vi "create and initialize.vi"(8 "error in":errorcluster, 10 "parameters":variant, 11 "function":T1) -> (0 "error out":errorcluster, 3 "call by reference action":refnum<class "call function by reference.lvclass">)   [LabVIEW 2014, in "call function by reference.lvclass"]
uses:
  call function by reference.lvclass
  function definition.ctl
  call function by reference.lvclass/call function by reference.ctl
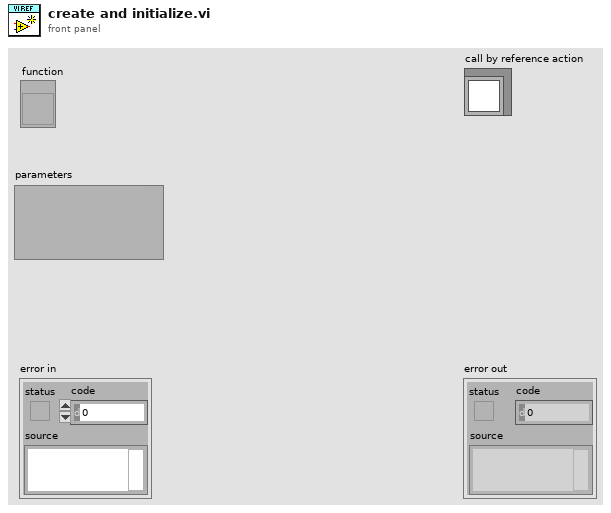
[diagram p1: front panel]
types:
  T1 = typedef "call function by reference.lvclass/function definition.ctl" = refnum<vi>
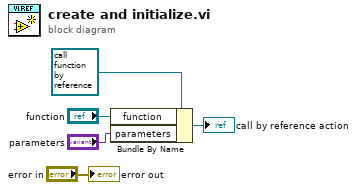
[diagram p0: block diagram]
diagram:
  n1 = Bundle By Name(cluster=refnum<class "call function by reference.lvclass"> refnum ("call by reference action in"), "function"="function", "parameters"="parameters") -> (→"call by reference action":refnum<class "call function by reference.lvclass">)
  "error out" <- "error in"
